vi "Create Identity Classes.vi"(9 "Classes":T1[](array[typedef]), 11 "Owning LVLib":refnum<vi>) -> (2 "Class Ref Map":variant, 3 "Owning LVLib Dup":refnum<vi>)   [LabVIEW 2013]
uses:
  Data Structures/JSON/Class.ctl
  Data Structures/JSON/Enum.ctl
  Data Structures/JSON/Enum Value.ctl
  Data Structures/JSON/Method.ctl
  Data Structures/JSON/Param.ctl
  Data Structures/JSON/Property.ctl
  Param Writers/TypeConv/Category.ctl
  Param Writers/TypeConv/Action.ctl
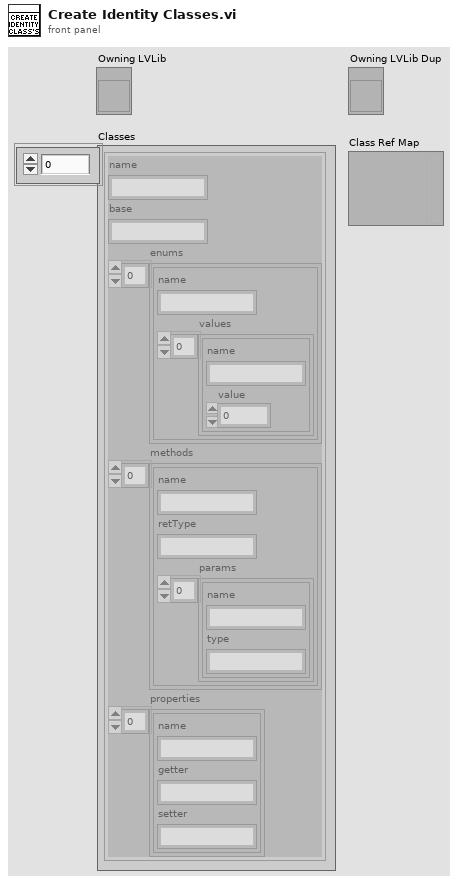
[diagram p1: front panel]
types:
  T1 = typedef "Class.ctl" = cluster{"name":string, "base":string, "enums":T2[], "methods":T4[], "properties":T6[]}
  T2 = typedef "Enum.ctl" = cluster{"name":string, "values":T3[]}
  T3 = typedef "Enum Value.ctl" = cluster{"name":string, "value":i32}
  T4 = typedef "Method.ctl" = cluster{"name":string, "retType":string, "params":T5[]}
  T5 = typedef "Param.ctl" = cluster{"name":string, "type":string}
  T6 = typedef "Property.ctl" = cluster{"name":string, "getter":string, "setter":string}
  T7 = typedef "Action.ctl" = enum16{"Register Type", "Obtain Writer"}
  T8 = typedef "Category.ctl" = enum16{"Invalid", "Void", "Boolean", "Numeric", "Enum", "SimpleStruct", "OpaqueStruct", "Identity", "SimpleContainer", "FullArray"}
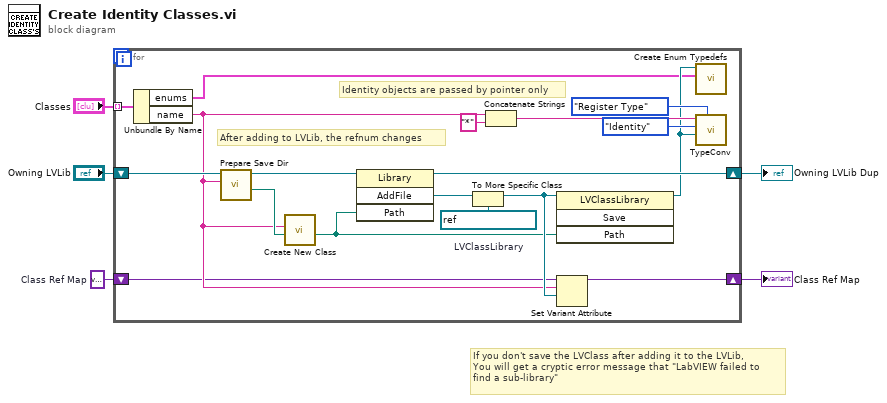
[diagram p0: block diagram]
diagram:
  w1 = variant  # Class Ref Map
  # "If you don't save the LVClass after adding it to the LVLib,\nYou will get a cryptic error message that \"LabVIEW failed to\nfind a sub-library\""
  n1 = for {
    shift-right: [w11] -> w3
    shift-left: "Owning LVLib" -> [w21]
    tunnel: "Classes" -> [w10] mode=indexing
    shift-right: [w17] -> w4
    shift-left: w1 -> [w8]
    w22 = refnum<vi> refnum  # LVClassLibrary
    # "Identity objects are passed by pointer only"
    # "After adding to LVLib, the refnum changes"
    n2 = Unbundle By Name(w10) -> ("enums"=w6:T2[], "name"=w9:string)
    n3 = call "Prepare Save Dir.vi"("Entity Name"=w9, "Owning LVLib"=w21) -> ("Entity Path"=w19:path, "Owning LVLib Dup"=w20:refnum<vi>)  [unwired: 8 in]
    n4 = call "Create New Class.vi"("Class Path"=w19, "Class Name"=w9) -> ("Class Path Dup"=w12:path)  [unwired: 8 in, 1 out]
    n5 = invoke class="Library" method="AddFile"(reference=w20, "Path"=w12) -> (reference out=w11:refnum<vi>, "AddFile"=w23:refnum<vi>)  [unwired: 2 in, 2 out]
    n6 = To More Specific Class(target class=w22, reference=w23) -> (specific class reference=w18:refnum<vi>)  [unwired: 1 in, 1 out]
    n7 = Concatenate Strings(w9, "*" ("string")) -> (w15:string)
    n8 = invoke class="LVClassLibrary" method="Save"(reference=w18, "Path"=w12) -> (reference out=w7:refnum<vi>)  [unwired: 2 in, 3 out]
    n9 = Set Variant Attribute(Variant=w8, name=w9, value=w18) -> (Variant out=w17:variant)  [unwired: 1 in, 2 out]
    n10 = call "Create Enum Typedefs.vi"("Enums"=w6, "Owning Lib"=w7) -> ()  [unwired: 9 in, 1 out]
    n11 = call "TypeConv.vi"("Action"=Action."Register Type", "LVClass Ref [Identity, OpaqueStruct]"=w7, "Category"=Category."Identity", "Type Name"=w15) -> ()  [unwired: 7 in, 1 out]
  }
  "Class Ref Map" <- w4
  "Owning LVLib Dup" <- w3
